vi "Apply Signal Names.vi"(8 "error in":errorcluster, 11 "SwitchMatrix in":refnum<class "SwitchMatrix.lvclass">) -> (0 "error out":errorcluster, 3 "SwitchMatrix out":refnum<class "SwitchMatrix.lvclass">)   [LabVIEW 2019, in "SwitchMatrix.lvlib" / "SwitchMatrix.lvclass"]
uses:
  SwitchMatrix.lvclass
  SwitchMatrix.lvclass/SwitchMatrix.ctl
  Accessors/Read Relay Name.vi
  Accessors/Read Configuration.vi
  Accessors/Write Relay Name.vi
  Accessors/Read Device.vi
  Desktop/Built/Configuration.lvlibp/Configuration.lvclass
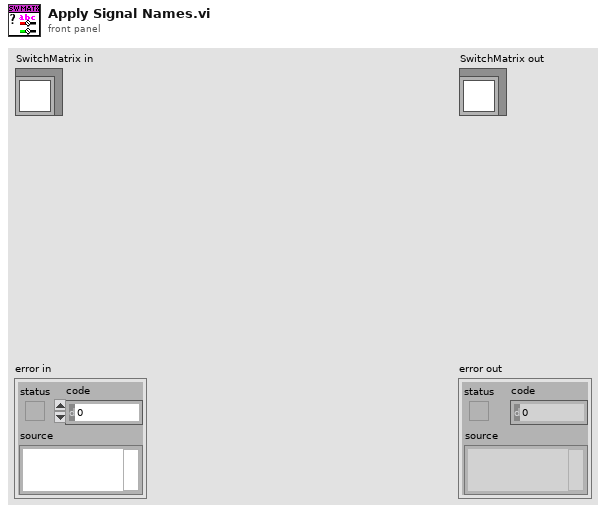
[diagram p1: front panel]
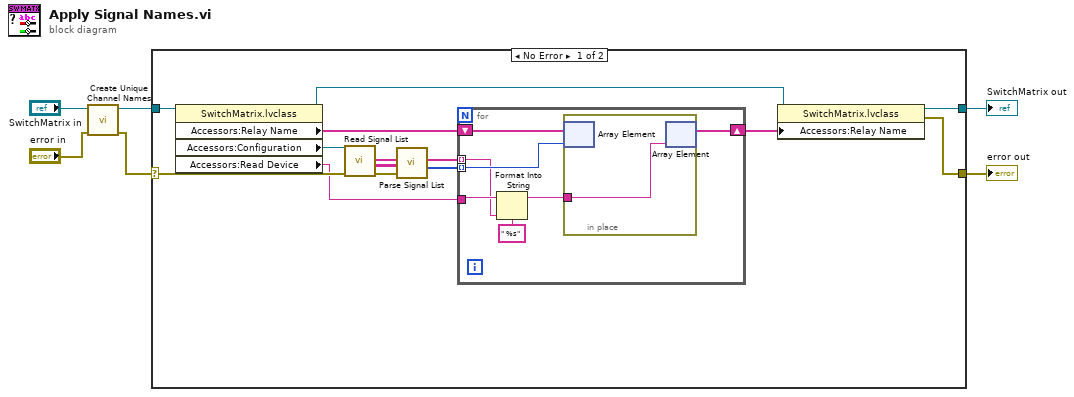
[diagram p0: block diagram]
diagram:
  n1 = call "Create Unique Channel Names.vi"("error in (no error)"="error in", "SwitchMatrix in"="SwitchMatrix in") -> ("error out"=w1:errorcluster, "SwitchMatrix out"=w3:refnum<class "SwitchMatrix.lvclass">)  [unwired: 8 in]
  n2 = case shown="No Error" w1 {
    selector: w1 -> [w17 w30]
    tunnel: [w12 w30] -> w6
    tunnel: [w13 w29] -> w5
    tunnel: w3 -> [w20 w29]
    frame No Error {
      n3 = property class="SwitchMatrix.lvclass"(reference=w20) -> (reference out=w18:refnum<class "SwitchMatrix.lvclass">, "Accessors:Relay Name"=w11:string[], "Accessors:Configuration"=w19:refnum<class "Configuration.lvclass">, "Accessors:Read Device"=w7:string)  [unwired: 1 in, 1 out]
      n4 = call "Read Signal List.vi"("error in (no error)"=w17, "Configuration in"=w19) -> ("error out"=w16:errorcluster, "Signal List"=w15:string[][], "Header"=w14:string[])  [unwired: 6 in, 1 out]
      n5 = call "Parse Signal List.vi"("error in"=w16, "Signal List"=w15, "Headers"=w14) -> ("Pins"=w8:i32[], "Names"=w9:string[])  [unwired: 6 in, 1 out]
      n6 = for {
        shift-right: [w26] -> w10
        shift-left: w11 -> [w27]
        tunnel: w9 -> [w22] mode=indexing
        tunnel: w8 -> [w25] mode=indexing
        tunnel: w7 -> [w24]
        n7 = Format Into String(format string=" %s", initial string=w24, w22) -> (resulting string=w21:string)  [unwired: 1 in, 1 out]
        n8 = in-place {
          in-place-border: w21 -> [w28]
          n9 = in-place-array #1(w27, w25) -> ()  [unwired: 1 out]
          n10 = in-place-array #1(w28) -> (w26:string[])  [unwired: 1 out]
        }
      }
      n11 = property class="SwitchMatrix.lvclass"(reference=w18, "Accessors:Relay Name"=w10) -> (reference out=w13:refnum<class "SwitchMatrix.lvclass">, error out=w12:errorcluster)  [unwired: 1 in]
    }
    frame Error {
    }
  }
  "error out" <- w6
  "SwitchMatrix out" <- w5
